vi "setWheelData_DriveQuadTalonSRX.vi"(6 "Time":T2, 7 "Distance Type":T1, 9 "Enc Edges / Rev":dbl=1440.0 format="%.4f", 10 "Gear Ratio":dbl=1.0 format="%.4f", 11 "Wheel Radius In":dbl=3.0 format="%.4f") -> (0 "VelUnits/Count in 0.1":dbl format="%.4f", 1 "Count/VelUnits In 0.1 SEC":dbl format="%.4f", 2 "Dist/Count":dbl format="%.4f", 3 "Count/Dist":dbl format="%.4f", 4 "Units":string)   [LabVIEW 2019, in "DriveQuadTalonSRX_Motor.lvlib"]
uses:
  DriveQuadTalonSRX_Motor.lvlib
  Time_Units_Control.ctl
  Dist_Type.ctl
  globals_DriveQuadTalonSRX.vi
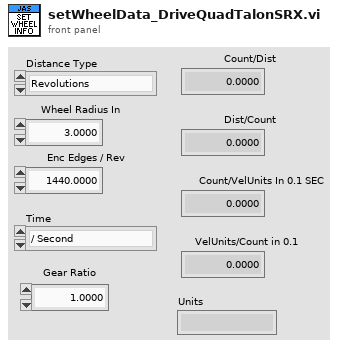
[diagram p1: front panel]
types:
  T1 = typedef "DriveQuadTalonSRX_Motor.lvlib/Dist_Type.ctl" = enum16{"Revolutions", "Feet"}
  T2 = typedef "DriveQuadTalonSRX_Motor.lvlib/Time_Units_Control.ctl" = enum16{"/ Second", "/ Minute"}
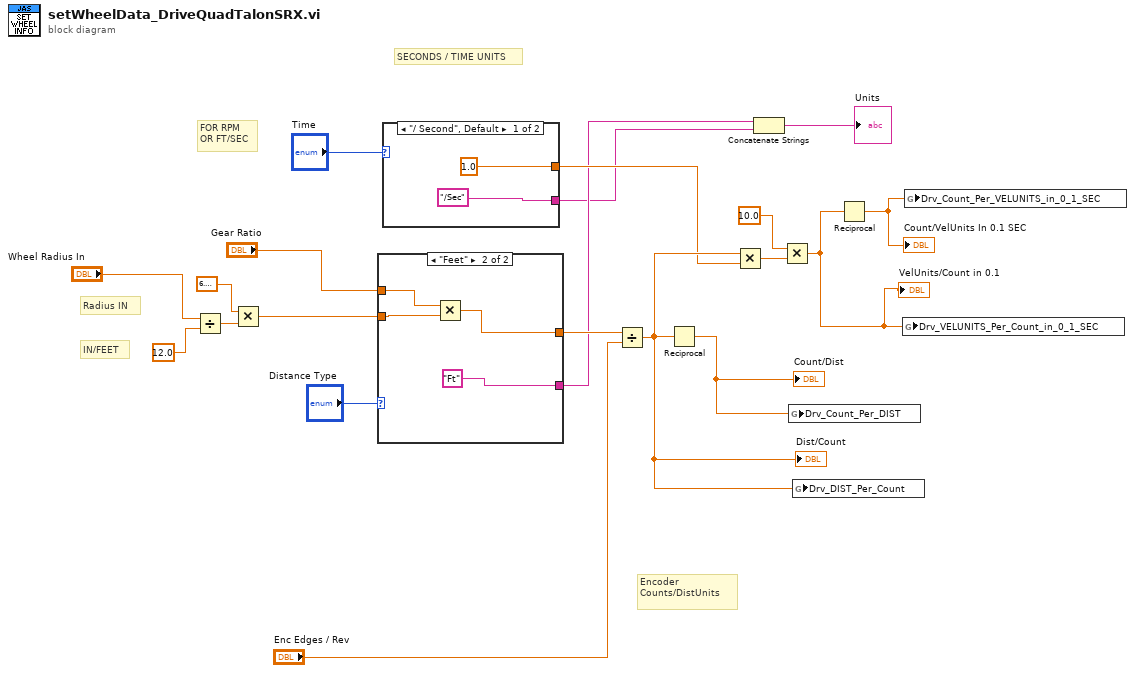
[diagram p0: block diagram]
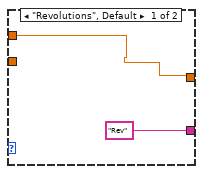
[diagram p2: hidden frame]
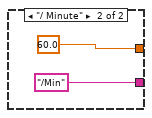
[diagram p3: hidden frame]
diagram:
  # "Encoder\nCounts/DistUnits"
  # "SECONDS / TIME UNITS"
  # "FOR RPM\nOR FT/SEC"
  # "IN/FEET"
  # "Radius IN"
  n1 = Divide(x="Wheel Radius In", y=12.0) -> (x/y=w16:dbl)
  n2 = Multiply(x=6.283185307179586, y=w16) -> (x*y=w11:dbl)
  n3 = case shown="\"Feet\"" "Distance Type" {
    tunnel: w11 -> [_ w25]
    tunnel: [w21 w23] -> w10
    tunnel: ["Rev" "Ft"] -> w6
    tunnel: "Gear Ratio" -> [w21 w24]
    frame "Revolutions", Default {
    }
    frame "Feet" {
      n4 = Multiply(x=w24, y=w25) -> (x*y=w23:dbl)
    }
  }
  n5 = case shown="\"/ Second\", Default" "Time" {
    tunnel: [1.0 60.0] -> w7
    tunnel: ["/Sec" "/Min"] -> w5
    frame "/ Second", Default {
    }
    frame "/ Minute" {
    }
  }
  n6 = Divide(x=w10, y="Enc Edges / Rev") -> (x/y=w8:dbl)
  "Dist/Count" <- w8
  n7 = Reciprocal(x=w8) -> (1/x=w20:dbl)
  "Count/Dist" <- w20
  n8 = Multiply(x=w8, y=w7) -> (x*y=w9:dbl)
  n9 = Concatenate Strings(w6, w5) -> (→"Units":string)
  n10 = Multiply(x=10.0 ("y"), y=w9) -> (x*y=w3:dbl)
  "VelUnits/Count in 0.1" <- w3
  n11 = global write "globals_DriveQuadTalonSRX.vi" "Drv_Count_Per_DIST"(w20) -> ()
  n12 = global write "globals_DriveQuadTalonSRX.vi" "Drv_DIST_Per_Count"(w8) -> ()
  n13 = Reciprocal(x=w3) -> (1/x=w2:dbl)
  "Count/VelUnits In 0.1 SEC" <- w2
  n14 = global write "globals_DriveQuadTalonSRX.vi" "Drv_VELUNITS_Per_Count_in_0_1_SEC"(w3) -> ()
  n15 = global write "globals_DriveQuadTalonSRX.vi" "Drv_Count_Per_VELUNITS_in_0_1_SEC"(w2) -> ()
